vi "ManualDelayStage.vi"() -> ()   [LabVIEW 2016]
uses:
  C:/Users/VaidaLabAdmin/Desktop/CodyEthanJordan/LaserControl/DelayStageDlls/Thorlabs.MotionControl.Controls.dll
  DelayStageDlls/Thorlabs.MotionControl.Controls.dll
  C:/Users/VaidaLabAdmin/Desktop/CodyEthanJordan/LaserControl/DelayStageDlls/Thorlabs.MotionControl.Benchtop.BrushlessMotorCLI.dll
  DelayStageDlls/Thorlabs.MotionControl.Benchtop.BrushlessMotorCLI.dll
  C:/Users/VaidaLabAdmin/Desktop/CodyEthanJordan/LaserControl/DelayStageDlls/Thorlabs.MotionControl.GenericMotorCLI.dll
  DelayStageDlls/Thorlabs.MotionControl.GenericMotorCLI.dll
panel:
  out "Rel. Position":dbl=10.990350000000001 format="%#_10g"
  in  "Go To":dbl=11.0
  in  "Home":dbl=11.0
  in  "Radio Buttons":enum32{"Stop", "Set Home", "Go to", "Position"}(radio)=enum."Position"
  in  "stop":bool
  in  "SerialNumber":string="73871558"
  in  "BenchtopBrushlessControl 2":refnum<k24>(container)
  # "Delay Stage"
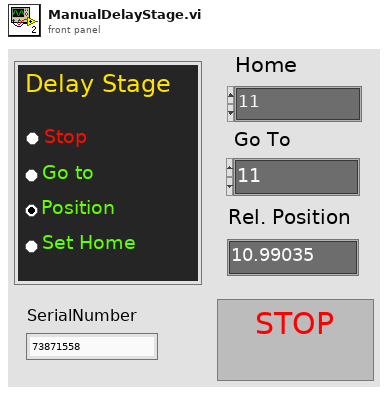
[diagram p1: front panel]
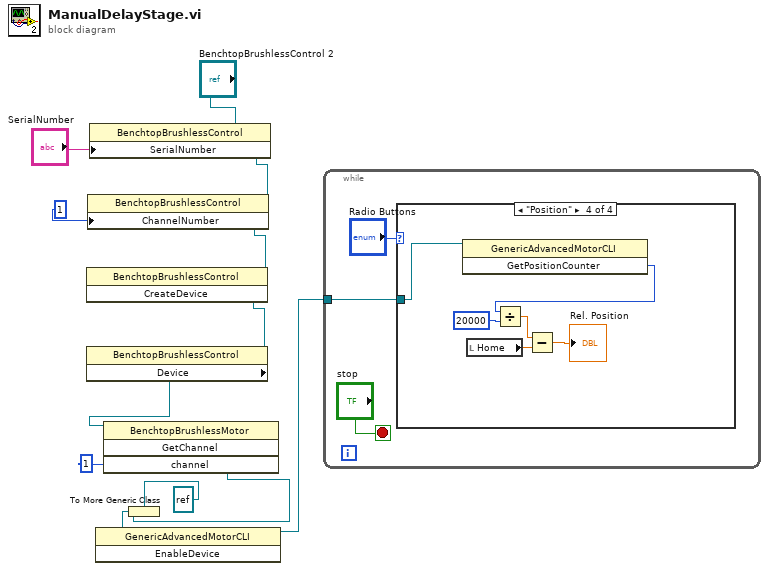
[diagram p0: block diagram]
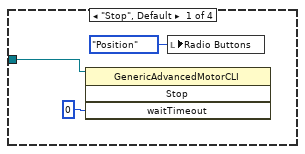
[diagram p2: hidden frame]
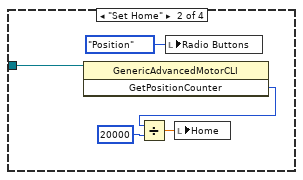
[diagram p3: hidden frame]
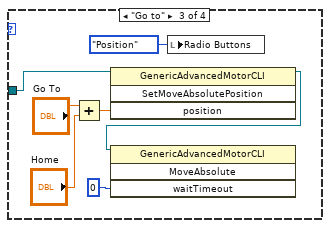
[diagram p4: hidden frame]
diagram:
  n1 = property class="BenchtopBrushlessControl"(reference="BenchtopBrushlessControl 2", "SerialNumber"="SerialNumber") -> (reference out=w8:refnum<k24>)  [unwired: 1 in, 1 out]
  n2 = property class="BenchtopBrushlessControl"(reference=w8, "ChannelNumber"=1) -> (reference out=w7:refnum<k24>)  [unwired: 1 in, 1 out]
  n3 = invoke class="BenchtopBrushlessControl" method="CreateDevice"(reference=w7) -> (reference out=w6:refnum<k24>)  [unwired: 2 in, 2 out]
  n4 = property class="BenchtopBrushlessControl"(reference=w6) -> ("Device"=w5:refnum<k24>)  [unwired: 1 in, 2 out]
  n5 = invoke class="BenchtopBrushlessMotor" method="GetChannel"(reference=w5, "channel"=i16 1) -> ("GetChannel"=w3:refnum<k24>)  [unwired: 2 in, 3 out]
  n6 = To More Generic Class(target class=refnum<k24> refnum, reference=w3) -> (generic class reference=w4:refnum<k24>)
  n7 = invoke class="GenericAdvancedMotorCLI" method="EnableDevice"(reference=w4) -> (reference out=w1:refnum<k24>)  [unwired: 2 in, 2 out]
  n8 = while {
    tunnel: w1 -> [w13]
    stop <- "stop" stop-if-true
    n9 = case shown="\"Position\"" "Radio Buttons" {
      tunnel: w13 -> [w16 w19 w25 w31]
      frame "Stop", Default {
        n10 = invoke class="GenericAdvancedMotorCLI" method="Stop"(reference=w16, "waitTimeout"=0) -> ()  [unwired: 2 in, 4 out]
        n11 = local write "Radio Buttons"(enum32{"Stop", "Set Home", "Go to", "Position"}."Position" ("Radio Buttons")) -> ()
      }
      frame "Set Home" {
        n12 = invoke class="GenericAdvancedMotorCLI" method="GetPositionCounter"(reference=w19) -> ("GetPositionCounter"=w22:i32)  [unwired: 2 in, 2 out]
        n13 = Divide(x=w22, y=20000) -> (x/y=w21:dbl)
        n14 = local write "Radio Buttons"(enum32{"Stop", "Set Home", "Go to", "Position"}."Position" ("Radio Buttons")) -> ()
        n15 = local write "Home"(w21) -> ()
      }
      frame "Go to" {
        n16 = Add(x="Go To", y="Home") -> (x+y=w28:dbl)
        n17 = invoke class="GenericAdvancedMotorCLI" method="SetMoveAbsolutePosition"(reference=w25, "position"=w28) -> (reference out=w26:refnum<k24>)  [unwired: 2 in, 3 out]
        n18 = invoke class="GenericAdvancedMotorCLI" method="MoveAbsolute"(reference=w26, "waitTimeout"=0) -> ()  [unwired: 2 in, 4 out]
        n19 = local write "Radio Buttons"(enum32{"Stop", "Set Home", "Go to", "Position"}."Position" ("Radio Buttons")) -> ()
      }
      frame "Position" {
        n20 = invoke class="GenericAdvancedMotorCLI" method="GetPositionCounter"(reference=w31) -> ("GetPositionCounter"=w35:i32)  [unwired: 2 in, 2 out]
        n21 = local read "Home"() -> (w32:dbl)
        n22 = Divide(x=w35, y=20000) -> (x/y=w34:dbl)
        n23 = Subtract(x=w34, y=w32) -> (x-y=→"Rel. Position":dbl)
      }
    }
  }
